vi "平化至XML.vi"() -> ()   [LabVIEW 2022 SP3]
doc: "本VI是为《我和LabVIEW》一书编写的示例。\n关于本书的介绍请参考网页：\nhttp://ruanqizhen.spaces.live.com/blog/cns!5852D4F797C53FB6!4310.entry"
panel:
  out "xml字符串":string
  out "值":dbl
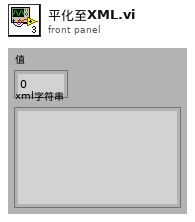
[diagram p1: front panel]
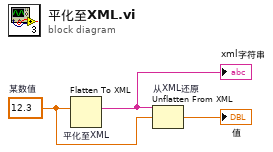
[diagram p0: block diagram]
diagram:
  w2 = 12.3  # 某数值
  n1 = Flatten To XML "平化至XML"(6:w2) -> (2:w3:string)
  "xml字符串" <- w3
  n2 = Unflatten From XML "从XML还原"(xml string=w3, type=w2) -> (value=→"值":dbl)  [unwired: 1 in, 1 out]
